vi "D_FlipFlop 1-1.vi"(2 "CLK":bool, 3 "D":bool) -> (0 "__\nQ":bool, 1 "Q":bool)   [LabVIEW 2018]
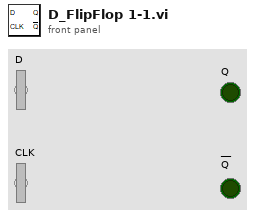
[diagram p1: front panel]
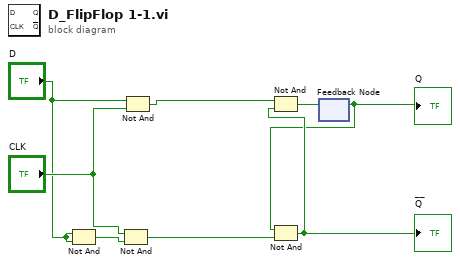
[diagram p0: block diagram]
diagram:
  n1 = Not And(1:"D", 2:"D") -> (0:w4:bool)
  n2 = Not And(1:w4, 2:"CLK") -> (0:w5:bool)
  n3 = Not And(1:"CLK", 2:"D") -> (0:w3:bool)
  n4 = feedback #1() -> (w6:bool)  [unwired: 1 in]
  "Q" <- w6
  n5 = Not And(1:w5, 2:w6) -> (0:w7:bool)
  "__\nQ" <- w7
  n6 = Not And(1:w7, 2:w3) -> (0:w8:bool)
  n7 = feedback-in #1(w8) -> ()
